vi "RSZVB Coercing Warning.vi"(7 "In Range?":bool, 8 "error in (no error)":errorcluster {"code" format="%.0x"}, 11 "VISA session":refnum<visa-resource-name>) -> (0 "error out":errorcluster {"code" format="%.0x"}, 3 "dup VISA session":refnum<visa-resource-name>)   [LabVIEW 2015]
doc: "This VI updates error cluster with an appropriate warning code (0x3FFC09F0) that user input has been coerced."
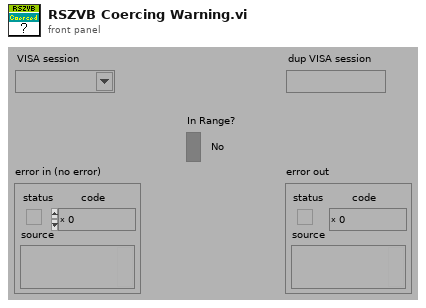
[diagram p1: front panel]
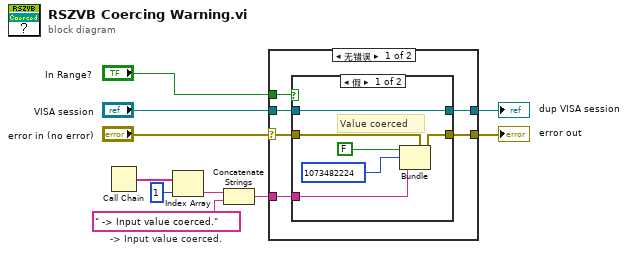
[diagram p0: block diagram]
diagram:
  w2 = " -> Input value coerced."  # -> Input value coerced.
  n1 = Call Chain() -> (call chain=w5:string[])
  n2 = Index Array(array=w5, index=1) -> (element=w3:string)
  n3 = Concatenate Strings(w3, w2) -> (w1:string)
  n4 = case shown="无错误" "error in (no error)" {
    selector: "error in (no error)" -> [w16 w25]
    tunnel: "VISA session" -> [w13 w26]
    tunnel: [w12 w26] -> w10
    tunnel: [w15 w25] -> w9
    tunnel: "In Range?" -> [w14 _]
    tunnel: w1 -> [w11 _]
    frame No Error {
      n5 = case shown="假" w14 {
        tunnel: w16 -> [w22 w24]
        tunnel: [w21 w24] -> w15
        tunnel: [w18 w23] -> w12
        tunnel: w13 -> [w18 w23]
        tunnel: w11 -> [w17 _]
        frame False {
          # "Value coerced"
          n6 = Bundle(cluster=w22, "status"=FALSE, "code"=1073482224, "source"=w17) -> (w21:errorcluster)
        }
        frame True {
        }
      }
    }
    frame Error {
    }
  }
  "error out" <- w9
  "dup VISA session" <- w10
